vi "FeedbackParameters.vi"(8 "error in":errorcluster, 9 "feedbackParameters":T1, 11 "FPGA VI Reference In":refnum<k20>) -> (0 "error out":errorcluster, 3 "FPGA VI Reference Out":refnum<k20>)   [LabVIEW 2016]
uses:
  <vilib>/rvi/errors/niLvFpgaAdjustHostInterfaceError.vi
  <vilib>/Utility/error.llb/Error Cluster From Error Code.vi
  <vilib>/rvi/interface/nirviReadWriteControl/nirviReadWriteControl.xnode
  NiFpgaLv.dll
  <vilib>/rvi/interface/Simulation/niFpgaSimulationCallBeginRW.vi
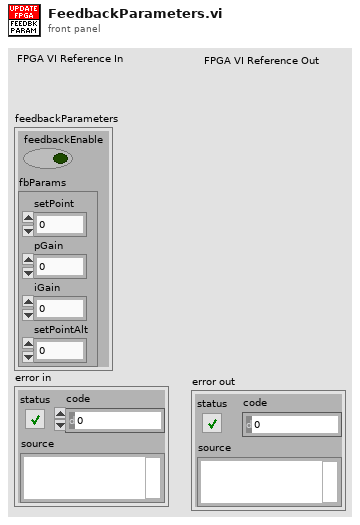
[diagram p1: front panel]
types:
  T1 = cluster{"feedbackEnable":bool, "fbParams":cluster{"setPoint":fxp<+/-,17,1>, "pGain":dbl, "iGain":dbl, "setPointAlt":fxp<+/-,17,1>}}
  T2 = cluster{"setPoint":fxp<+/-,17,1>, "pGain":fxp<+/-,20,1>, "iGain":fxp<+/-,20,1>, "gainScale":i8}
  T3 = cluster{"setPoint":fxp<+/-,17,1>, "pGain":dbl, "iGain":dbl, "setPointAlt":fxp<+/-,17,1>}
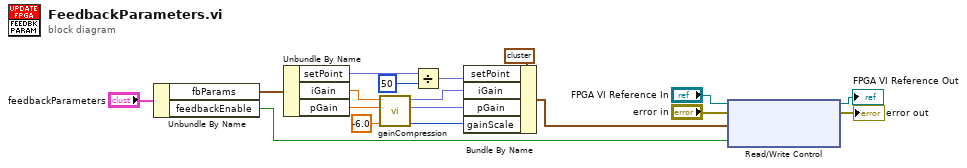
[diagram p0: block diagram]
diagram:
  n1 = Unbundle By Name("feedbackParameters") -> ("fbParams"=w12:T3, "feedbackEnable"=w7:bool)
  n2 = Unbundle By Name(w12) -> ("setPoint"=w10:fxp<+/-,17,1>, "iGain"=w17:dbl, "pGain"=w18:dbl)
  n3 = call "gainCompression.vi"("compressionMin"=-6.0, "slaveInput"=w18, "masterInput"=w17) -> ("gainScale"=w14:i8, "rescaledSlave"=w15:fxp<+/-,20,1>, "rescaledMaster"=w16:fxp<+/-,20,1>)  [unwired: 6 in]
  n4 = Divide(x=w10, y=50) -> (x/y=w11:fxp<+/-,50,2>)
  n5 = Bundle By Name(cluster=T2 {"setPoint"=0.0, "pGain"=0.0, "iGain"=0.0, "gainScale"=0} ("feedbackbParams"), "setPoint"=w11, "iGain"=w16, "pGain"=w15, "gainScale"=w14) -> (w2:T2)
  n6 = xnode "Read/Write Control"("FPGA VI Reference In"="FPGA VI Reference In", "error in"="error in", "feedbackbParams"=w2, "enableFeedback"=w7) -> ("FPGA VI Reference Out"=→"FPGA VI Reference Out":refnum<k20>, "error out"=→"error out":errorcluster)
